vi "Bundle Script_Terminal Property or Method.vi"(6 "Object Placement":enum32{"Choice 1", "Choice 2"}(radio), 7 "Action":T1, 8 "error in":errorcluster, 9 "Property Array":T3(array[cluster]), 11 "Affected Items":T2) -> (0 "error out":errorcluster, 2 "Objects":refnum<vi>[](array[refnum]))   [LabVIEW 2023]
doc: "Wire invoke or property node to terminal."
uses:
  top/BundleMagic.ctl
  controls/action enum.ctl
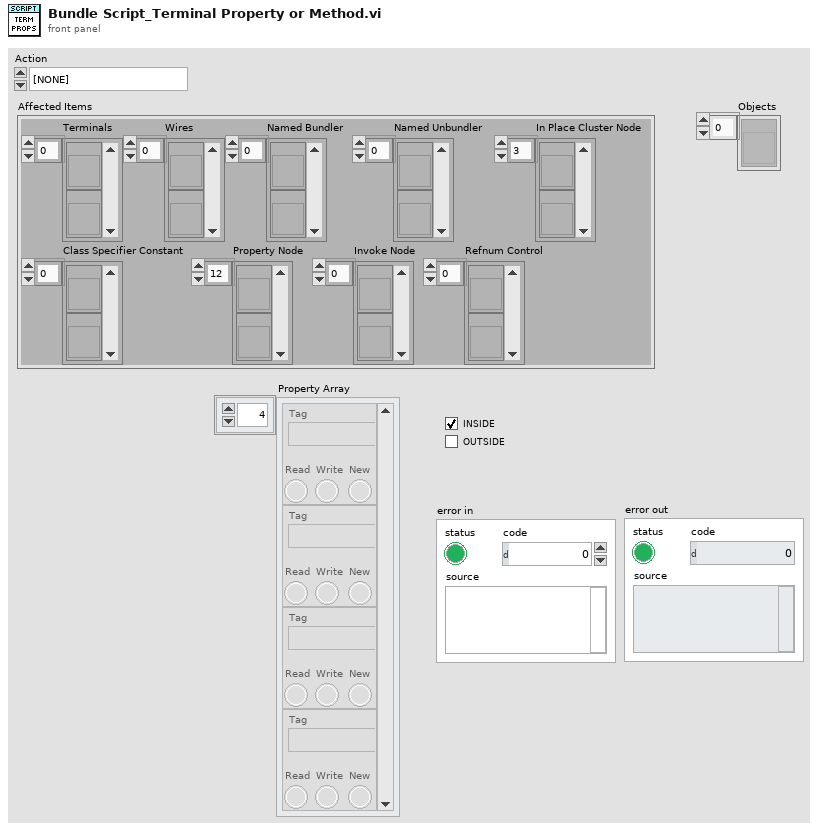
[diagram p1: front panel]
types:
  T1 = typedef "action enum.ctl" = enum16{"[NONE]", "Wire Bundle", "Wire Unbundle", "Terminal Unbundle", "Terminal Bundle", "Bundler Move Up", "Bundler Move Down", "Bundler Insert", "Bundler Remove", "Bundler Remove Unwired", "Bundler Rearrange", "In Place Insert", "In Place Remove", "In Place Remove Unwired", "In Place Rearrange", "Wire Properties", "Wire Method", "Terminal Properties", "Terminal Method", "Property Move Up", "Property Move Down", "Properties Insert", "Properties Remove", "Properties Remove Unwired", "Properties Rearrange", "Method Change", "Class for Constant", "Class For Control", "Class For Node", "Class Name to Clipboard"}
  T2 = typedef "BundleMagic.ctl" = cluster{"Terminals":refnum<vi>[], "Wires":refnum<vi>[], "Named Bundler":refnum<vi>[], "Named Unbundler":refnum<vi>[], "In Place Cluster Node":refnum<vi>[], "Class Specifier Constant":refnum<vi>[], "Property Node":refnum<vi>[], "Invoke Node":refnum<vi>[], "Refnum Control":refnum<vi>[]}
  T3 = cluster{"Tag":string, "Read":bool, "Write":bool, "New":bool}[]
  T4 = cluster{"Tunnel Ref":refnum<vi>, "On Tunnel?":bool, "Placement":enum32{"Choice 1", "Choice 2"}, "Tunnel Is Indexing?":bool, "Diagram":refnum<vi>, "Position":cluster{"Refnum":refnum<vi>, "Relative Direction":enum32{"Right", "Left", "Top", "Bottom", "Top Right", "Top Left", "Bottom Right", "Bottom Left"}, "Point32":cluster{"Horizontal":i32, "Vertical":i32}}, "Chosen Terminal":refnum<vi>, "Is Refnum?":bool, "Is Cluster?":bool, "Is Source?":bool, "Tunnel Direction":enum16{"In-Going", "Out-Going"}, "Tunnel Position":enum16{"Left", "Top", "Right", "Bottom"}, "Is Inner?":bool, "Terminal Is Indexing?":bool}
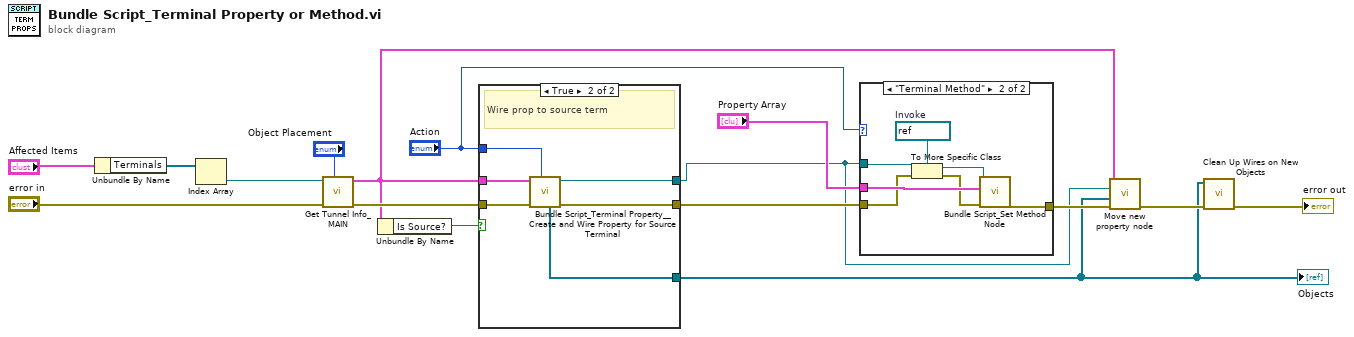
[diagram p0: block diagram]
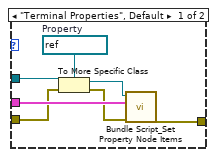
[diagram p2: hidden frame]
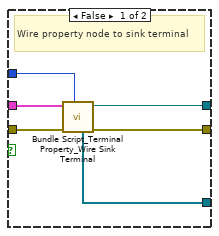
[diagram p3: hidden frame]
diagram:
  n1 = Unbundle By Name("Affected Items") -> ("Terminals"=w10:refnum<vi>[])
  n2 = Index Array(array=w10) -> (element=w11:refnum<vi>)  [unwired: 1 in]
  n3 = call "Get Tunnel Info_MAIN.vi"("Object Placement"="Object Placement", "error in"="error in", "Terminal in"=w11) -> ("error out"=w14:errorcluster, "Terminal Data Cluster"=w4:T4)  [unwired: 6 in, 1 out]
  n4 = Unbundle By Name(w4) -> ("Is Source?"=w13:bool)
  n5 = case shown="True" w13 {
    tunnel: [w19 w25] -> w15
    tunnel: w14 -> [w21 w27]
    tunnel: [w20 w24] -> w1
    tunnel: [w18 w26] -> w3
    tunnel: w4 -> [w22 w28]
    tunnel: "Action" -> [w17 w23]
    frame False {
      # "Wire property node to sink terminal"
      n6 = call "Bundle Script_Terminal Property_Wire Sink Terminal.vi"("Action"=w17, "error in"=w21, "Terminal Data Cluster"=w22) -> ("error out"=w19:errorcluster, "New Node Refnum"=w20:refnum<vi>, "New objects created"=w18:refnum<vi>[])  [unwired: 6 in]
    }
    frame True {
      # "Wire prop to source term"
      n7 = call "Bundle Script_Terminal Property__Create and Wire Property for Source Terminal.vi"("Action"=w23, "error in"=w27, "Terminal Data Cluster"=w28) -> ("error out"=w25:errorcluster, "Property Refnum"=w24:refnum<vi>, "New objects created"=w26:refnum<vi>[])  [unwired: 6 in]
    }
  }
  "Objects" <- w3
  n8 = case shown="\"Terminal Method\"" "Action" {
    tunnel: w15 -> [w29 w36]
    tunnel: "Property Array" -> [w35 w42]
    tunnel: [w34 w41] -> w6
    tunnel: w1 -> [w33 w40]
    frame "Terminal Properties", Default {
      w31 = refnum<vi> refnum  # Property
      n9 = To More Specific Class(target class=w31, reference=w33, error in=w29) -> (specific class reference=w32:refnum<vi>, error out=w30:errorcluster)
      n10 = call "Bundle Script_Set Property Node Items.vi"("error in"=w30, "Property Array"=w35, "Property Node Ref"=w32) -> ("error out"=w34:errorcluster)  [unwired: 8 in]
    }
    frame "Terminal Method" {
      w39 = refnum<vi> refnum  # Invoke
      n11 = To More Specific Class(target class=w39, reference=w40, error in=w36) -> (specific class reference=w38:refnum<vi>, error out=w37:errorcluster)
      n12 = call "Bundle Script_Set Method Node.vi"("error in"=w37, "Property Array"=w42, "Invoke in"=w38) -> ("error out"=w41:errorcluster)  [unwired: 8 in]
    }
  }
  n13 = call "Move new property node.vi"("error in"=w6, "New objects created"=w3, "Property Node Ref"=w1, "Terminal Data Cluster"=w4) -> ("error out"=w5:errorcluster)  [unwired: 7 in]
  n14 = call "Clean Up Wires on New Objects.vi"("error in (no error)"=w5, "New objects created"=w3) -> ("error out"=→"error out":errorcluster)  [unwired: 9 in]
